vi "Find Referenced Structure in Tree.vi"(8 "error in":errorcluster, 10 "SNAME":string, 11 "ParseGDSII in":refnum<class "ParseGDSII.lvclass">) -> (0 "error out":errorcluster, 2 "Structure Nodes":T1, 3 "ParseGDSII out":refnum<class "ParseGDSII.lvclass">)   [LabVIEW 2019, in "ParseGDSII.lvclass"]
uses:
  ParseGDSII.lvclass
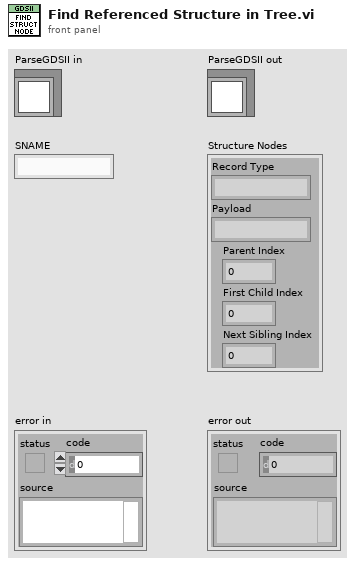
[diagram p1: front panel]
types:
  T1 = cluster{"Record Type":string, "Payload":string, "Parent Index":i32, "First Child Index":i32, "Next Sibling Index":i32}
  T2 = cluster{"Record Type":string, "Payload":string, "Parent Index":i32, "First Child Index":i32, "Next Sibling Index":i32}[]
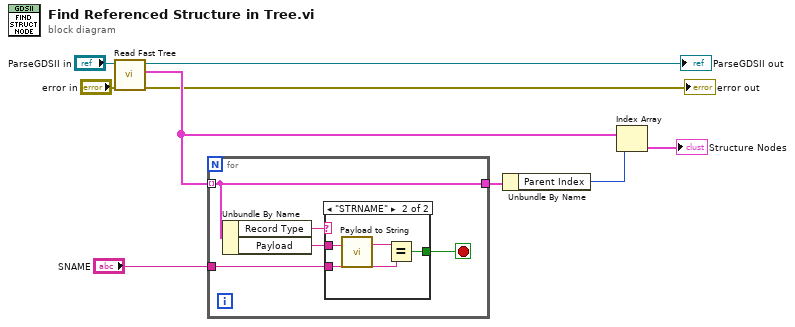
[diagram p0: block diagram]
diagram:
  n1 = call "Read Fast Tree.vi"("error in"="error in", "ParseGDSII in"="ParseGDSII in") -> ("error out"=→"error out":errorcluster, "Tree"=w7:T2, "ParseGDSII out"=→"ParseGDSII out":refnum<class "ParseGDSII.lvclass">)  [unwired: 6 in, 1 out]
  n2 = for {
    tunnel: w7 -> [w11] mode=indexing
    tunnel: "SNAME" -> [w13]
    tunnel: [w11] -> w9
    stop <- w10 stop-if-true
    n3 = Unbundle By Name(w11) -> ("Record Type"=w14:string, "Payload"=w12:string)
    n4 = case shown="\"STRNAME\"" w14 {
      tunnel: w13 -> [_ w16]
      tunnel: w12 -> [_ w18]
      tunnel: [_ w15] -> w10
      frame "False", Default {
      }
      frame "STRNAME" {
        n5 = call "Payload to String.vi"("Payload"=w18) -> ("String"=w17:string)  [unwired: 2 in]
        n6 = Equal?(x=w17, y=w16) -> (x = y?=w15:bool)
      }
    }
  }
  n7 = Unbundle By Name(w9) -> ("Parent Index"=w8:i32)
  n8 = Index Array(array=w7, index=w8) -> (element=→"Structure Nodes":T1)
